vi "INTELLIFAUCET Valve Hold.vi"(6 "MW100 Sema":T1, 8 "error in (no error)":errorcluster, 11 "VISA Refnum in":refnum<visa-resource-name>) -> (0 "error out":errorcluster, 3 "VISA Refnum out":refnum<visa-resource-name>)   [LabVIEW 2016]
uses:
  Type Definitions/INTELLIFAUCET Set Mode.ctl
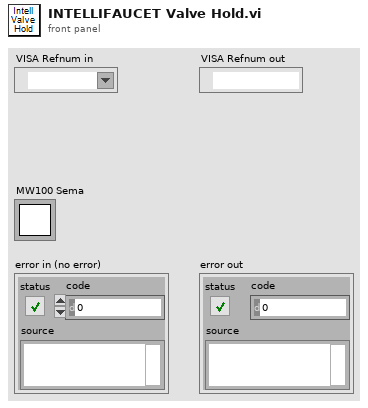
[diagram p1: front panel]
types:
  T1 = typedef "Semaphore RefNum" = refnum<k1>
  T2 = typedef "INTELLIFAUCET Set Mode.ctl" = enum16{"Adjust Temp", "Adjust Flow", "Start Flow", "Stop Flow", "Hold"}
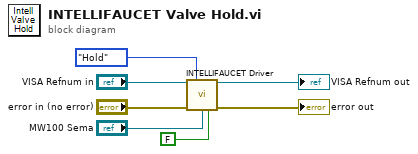
[diagram p0: block diagram]
diagram:
  n1 = call "INTELLIFAUCET Driver.vi"("VISA session"="VISA Refnum in", "Mode"=INTELLIFAUCET_Set_Mode."Hold", "Error In"="error in (no error)", "Refnum in"="MW100 Sema", "Use Proportion Valve"=FALSE) -> ("VISA session out"=→"VISA Refnum out":refnum<visa-resource-name>, "Error Out"=→"error out":errorcluster)  [unwired: 7 in, 2 out]
